vi "Get_Notifier.vi"(2 "error in":errorcluster, 3 "name":string="ImagingSynch") -> (0 "error out":errorcluster)   [LabVIEW 2012]
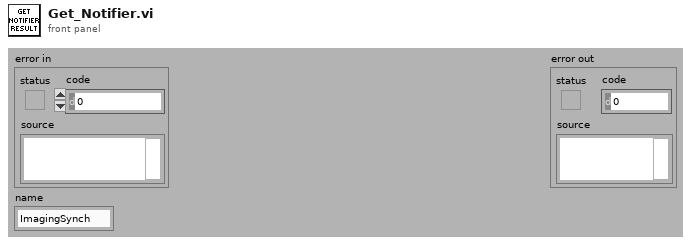
[diagram p1: front panel]
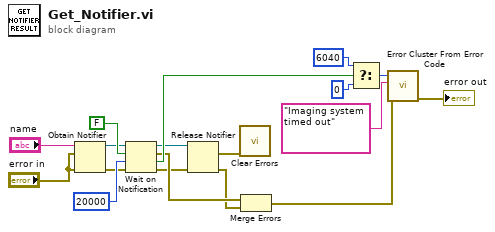
[diagram p0: block diagram]
diagram:
  n1 = Obtain Notifier(name (unnamed)="name", notification data type="error in", error in (no error)="error in") -> (notifier out=w14:refnum<notifier>, error out=w13:errorcluster)  [unwired: 1 in, 1 out]
  n2 = Wait on Notification(notifier=w14, ignore previous (F)=FALSE, timeout in ms (-1)=20000, error in (no error)=w13) -> (notifier out=w4:refnum<notifier>, notification=w6:errorcluster, timed out?=w12:bool, error out=w3:errorcluster)
  n3 = Release Notifier(notifier=w4, error in (no error)=w3) -> (last notification=w1:errorcluster, error out=w2:errorcluster)  [unwired: 1 in, 1 out]
  n4 = call <vilib>:"Clear Errors.vi"("error in (no error)"=w1) -> ()  [unwired: 6 in, 1 out]
  n5 = Merge Errors(w6, w2) -> (w7:errorcluster)
  n6 = Select(t=6040, s=w12, f=0 ("error code (0)")) -> (s? t:f=w9:i32)
  n7 = call <vilib>:"Error Cluster From Error Code.vi"("error in (no error)"=w7, "error message (\"\")"="Imaging system timed out" ("error message (\"\")"), "error code (0)"=w9) -> ("error out"=→"error out":errorcluster)  [unwired: 6 in]
